vi "LED_Control_NN.vi"() -> ()   [LabVIEW 2022 SP3]
panel:
  in  "stop":bool
  in  "VISA resource name":refnum<visa-resource-name>
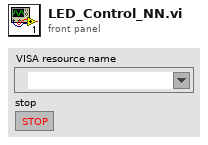
[diagram p1: front panel]
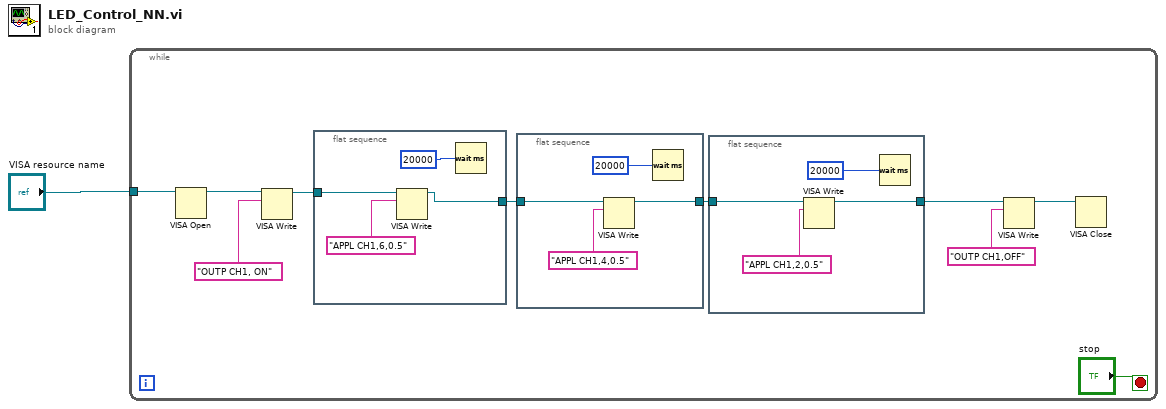
[diagram p0: block diagram]
diagram:
  n1 = while {
    tunnel: "VISA resource name" -> [w3]
    stop <- "stop" stop-if-true
    n2 = VISA Open(VISA resource name=w3) -> (VISA resource name=w11:refnum<visa-resource-name>)  [unwired: 4 in, 1 out]
    n3 = VISA Write(VISA resource name=w11, write buffer="OUTP CH1, ON") -> (VISA resource name out=w9:refnum<visa-resource-name>)  [unwired: 1 in, 2 out]
    n4 = flat-sequence {
      tunnel: w9 -> [w21]
      tunnel: [w20] -> w8
      frame #0 {
        n5 = VISA Write(VISA resource name=w21, write buffer="APPL CH1,6,0.5") -> (VISA resource name out=w20:refnum<visa-resource-name>)  [unwired: 1 in, 2 out]
        n6 = Wait (ms)(milliseconds to wait=20000) -> ()  [unwired: 1 out]
      }
    }
    n7 = flat-sequence {
      tunnel: w8 -> [w17]
      tunnel: [w16] -> w7
      frame #0 {
        n8 = VISA Write(VISA resource name=w17, write buffer="APPL CH1,4,0.5") -> (VISA resource name out=w16:refnum<visa-resource-name>)  [unwired: 1 in, 2 out]
        n9 = Wait (ms)(milliseconds to wait=20000) -> ()  [unwired: 1 out]
      }
    }
    n10 = flat-sequence {
      tunnel: w7 -> [w13]
      tunnel: [w12] -> w6
      frame #0 {
        n11 = VISA Write(VISA resource name=w13, write buffer="APPL CH1,2,0.5") -> (VISA resource name out=w12:refnum<visa-resource-name>)  [unwired: 1 in, 2 out]
        n12 = Wait (ms)(milliseconds to wait=20000) -> ()  [unwired: 1 out]
      }
    }
    n13 = VISA Write(VISA resource name=w6, write buffer="OUTP CH1,OFF") -> (VISA resource name out=w5:refnum<visa-resource-name>)  [unwired: 1 in, 2 out]
    n14 = VISA Close(VISA resource name=w5) -> ()  [unwired: 1 in, 1 out]
  }
